vi "CANOpen SDOs - startup.vi"(8 "error in (no error)":errorcluster, 11 "Node Ptr":T2 format="%.0x") -> (0 "error out":errorcluster)   [LabVIEW 2013, in "CANOpen Addon Custom Device.lvlib"]
uses:
  CANOpen Addon Custom Device.lvlib
  <vilib>/NI Veristand/Custom Device API/Custom Device Item Ref.ctl
  SubVIs/CANOpen_SDO data format.ctl
  Shared Code/CANOpen_SDO Settings.ctl
  Shared Code/CANOpen Addon GUID Lookup Global.vi
  <vilib>/NI Veristand/Custom Device API/Get Item Property (Variant).vi
  <vilib>/NI Veristand/Custom Device API/Custom Device API.lvlib
panel:
  in  "Display format":T1
  out "SDOs":i32(listbox)
  in  "SHDocVw.IWebBrowser2":refnum<k7>(container)
  in  "Header":cluster{"Section Name":string}={"Section Name"="SDOs"}
  in  "Description":string
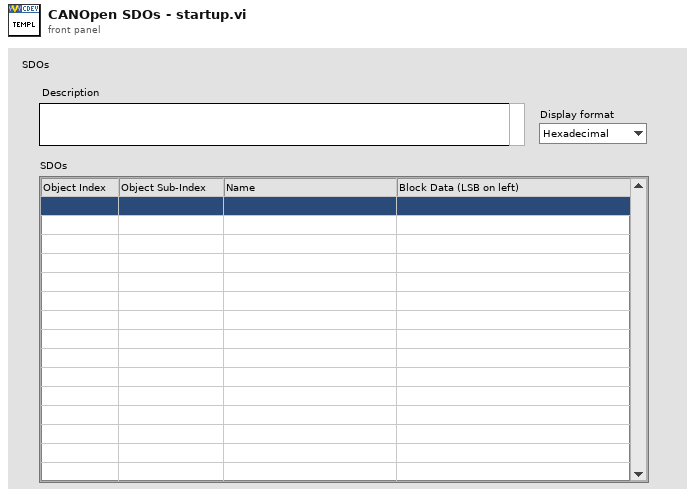
[diagram p1: front panel]
types:
  T1 = typedef "CANOpen Addon Custom Device.lvlib/CANOpen_SDO data format.ctl" = enum16{"Hexadecimal", "Decimal"}
  T2 = typedef "Custom Device API.lvlib/Custom Device Item Ref.ctl" = u64
  T3 = typedef "CANOpen Addon Custom Device.lvlib/CANOpen_SDO Settings.ctl" = cluster{"Object Index":u16, "Sub-Index (0)":u8, "Block Data":u8[], "Name":string}
  T4 = typedef "Custom Device API.lvlib/Custom Device Commands.ctl" = enum16{"Default", "Item renamed", "Shutdown", "Dynamic button pressed"}
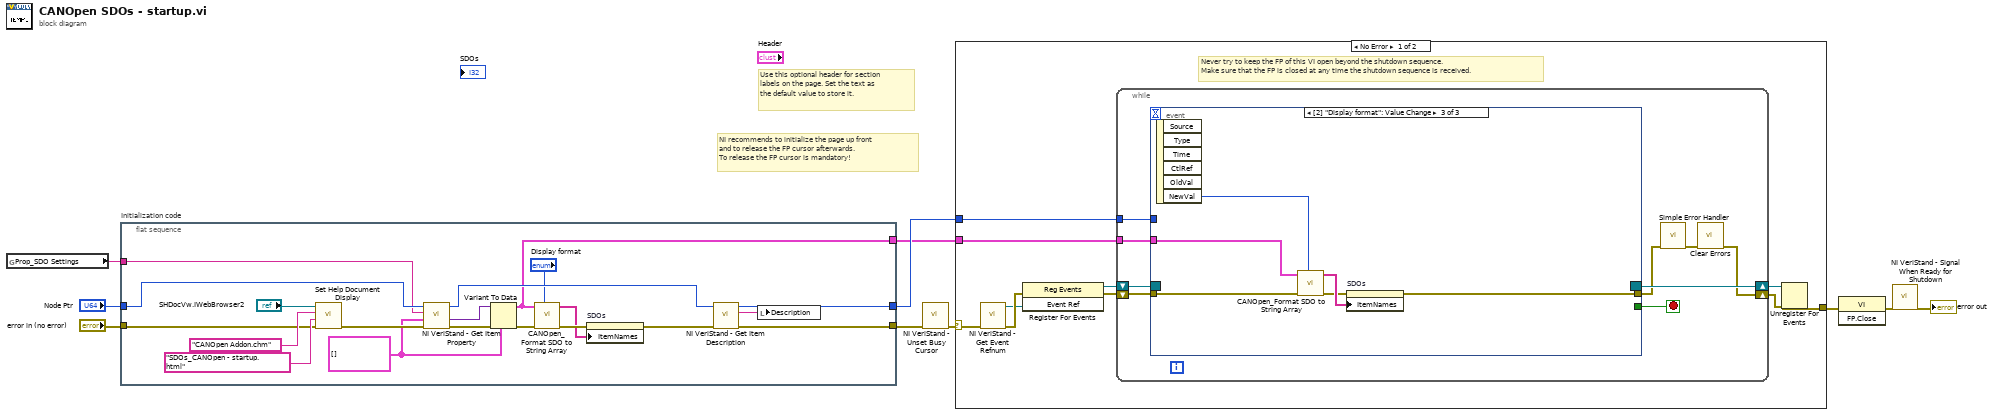
[diagram p0: block diagram]
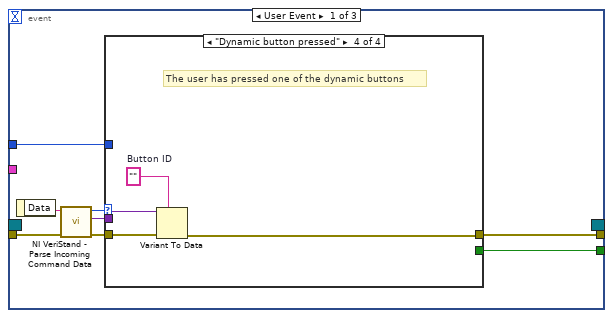
[diagram p2: hidden frame]
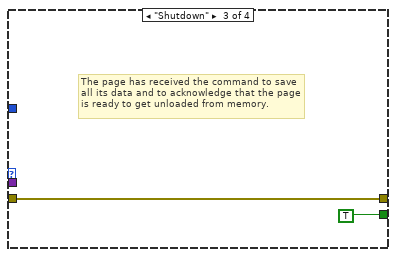
[diagram p5: hidden frame]
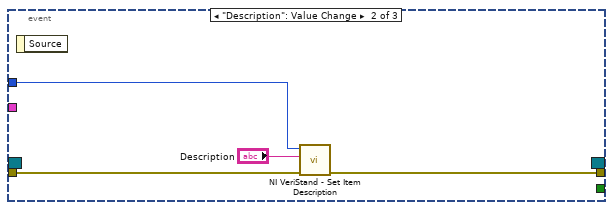
[diagram p6: hidden frame]
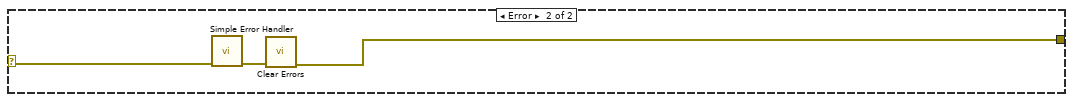
[diagram p7: hidden frame]
diagram:
  # "Use this optional header for section labels on the page. Set the text as the default value to store it."
  # "NI recommends to initialize the page up front\nand to release the FP cursor afterwards.\nTo release the FP cursor is mandatory!"
  n1 = global read "CANOpen Addon GUID Lookup Global.vi" "Prop_SDO Settings"() -> (w2:string)
  n2 = flat-sequence "Initialization code" {
    tunnel: "error in (no error)" -> [w26]
    tunnel: "Node Ptr" -> [w24]
    tunnel: [w13] -> w6
    tunnel: [w12] -> w3
    tunnel: w2 -> [w22]
    tunnel: [w11] -> w1
    frame #0 {
      w19 = T3[] [] ("SDO Parameters")
      n3 = call "Set Help Document Display.vi"("error in (no error)"=w26, "HTML File"="SDOs_CANOpen - startup.html", "Main CHM File"="CANOpen Addon.chm", "SHDocVw.IWebBrowser2"="SHDocVw.IWebBrowser2") -> ("error out"=w25:errorcluster)  [unwired: 7 in]
      n4 = call-poly <vilib>:"NI VeriStand - Get Item Property.vi"("error in (no error)"=w25, "Default Value"=w19, "Property Name"=w22, "Item Ref in"=w24) -> ("error out"=w21:errorcluster, "Value"=w20:variant, "Item Ref out"=w23:T2)  [unwired: 4 in, 1 out]
      n5 = Variant To Data(error in=w21, type=w19, Variant=w20) -> (data=w11:T3[], error out=w18:errorcluster)
      n6 = call "CANOpen_Format SDO to String Array.vi"("Format"="Display format", "error in (no error)"=w18, "SDO Parameters"=w11) -> ("error out"=w17:errorcluster, "Array"=w15:string[][])  [unwired: 7 in]
      n7 = property on="SDOs" class="MCListbox (strict)"(error in=w17, "ItemNames"=w15) -> (error out=w16:errorcluster)  [unwired: 1 in, 1 out]
      n8 = call <vilib>:"NI VeriStand - Get Item Description.vi"("error in (no error)"=w16, "Item Ref in"=w23) -> ("error out"=w13:errorcluster, "Description"=w30:string, "Item Ref out"=w12:T2)  [unwired: 7 out]
      n9 = local write "Description"(w30) -> ()
    }
  }
  n10 = call <vilib>:"NI VeriStand - Unset Busy Cursor.vi"("error in (no error)"=w6) -> ("error out"=w5:errorcluster)  [unwired: 10 out]
  n11 = case shown="No Error" w5 {
    selector: w5 -> [w32 w78]
    tunnel: [w37 w76] -> w10
    tunnel: w3 -> [w33 _]
    tunnel: w1 -> [w31 _]
    frame No Error {
      # "Never try to keep the FP of this VI open beyond the shutdown sequence.\nMake sure that the FP is closed at any time the shutdown sequence is received."
      n12 = call <vilib>:"NI VeriStand - Get Event Refnum.vi"("error in (no error)"=w32) -> ("error out"=w40:errorcluster, "Event Ref"=w36:refnum<user-event>)  [unwired: 9 out]
      n13 = register-events(error in=w40, w36) -> (reference out=w34:refnum<event-registration>, error out=w35:errorcluster)  [unwired: 1 in]
      n14 = while {
        tunnel: w33 -> [w45]
        shift-right: [w42] -> w38
        shift-left: w35 -> [w48]
        shift-right: [w49] -> w39
        shift-left: w34 -> [w47]
        tunnel: w31 -> [w41]
        stop <- w46 stop-if-true
        n15 = event shown="[2] \"Display format\": Value Change" {
          selector: w47 -> [_ _ _]
          dyn-events: [_ _ _] -> w49
          timeout: _ -> [_ _ _]
          tunnel: w48 -> [w57 w68 w71]
          tunnel: [w53 _ _] -> w46
          tunnel: [w52 w67 w70] -> w44
          tunnel: w45 -> [w51 w69 _]
          tunnel: w41 -> [_ _ w73]
          event User Event {
            n16 = event-data() -> ("Data"=w56:string)  [unwired: 1 out]
            n17 = call <vilib>:"NI VeriStand - Parse Incoming Command Data.vi"("error in (no error)"=w57, "Incoming data"=w56) -> ("error out"=w55:errorcluster, "Outgoing data"=w50:variant, "Action"=w54:T4)  [unwired: 7 out]
            n18 = case shown="\"Dynamic button pressed\"" w54 {
              tunnel: w55 -> [w58 w59 w60 w65]
              tunnel: [_ _ TRUE _] -> w53
              tunnel: [w58 w59 w60 w62] -> w52
              tunnel: w51 -> [_ _ _ _]
              tunnel: w50 -> [_ _ _ w64]
              frame "Default", Default {
              }
              frame "Item renamed" {
              }
              frame "Shutdown" {
                # "The page has received the command to save all its data and to acknowledge that the page is ready to get unloaded from memory."
              }
              frame "Dynamic button pressed" {
                w63 = ""  # Button ID
                # "The user has pressed one of the dynamic buttons"
                n19 = Variant To Data(error in=w65, type=w63, Variant=w64) -> (error out=w62:errorcluster)  [unwired: 1 out]
              }
            }
          }
          event "Description": Value Change {
            n20 = event-data() -> ()  [unwired: 2 out]
            n21 = call <vilib>:"NI VeriStand - Set Item Description.vi"("error in (no error)"=w68, "Description"="Description", "Item Ref in"=w69) -> ("error out"=w67:errorcluster)  [unwired: 8 out]
          }
          event Value Change {
            n22 = event-data() -> ("NewVal"=w72:T1)  [unwired: 6 out]
            n23 = call "CANOpen_Format SDO to String Array.vi"("Format"=w72, "error in (no error)"=w71, "SDO Parameters"=w73) -> ("error out"=w74:errorcluster, "Array"=w75:string[][])  [unwired: 7 in]
            n24 = property on="SDOs" class="MCListbox (strict)"(error in=w74, "ItemNames"=w75) -> (error out=w70:errorcluster)  [unwired: 1 in, 1 out]
          }
        }
        n25 = call <vilib>:"Simple Error Handler.vi"("error in (no error)"=w44) -> ("error out"=w43:errorcluster)  [unwired: 1 in, 7 out]
        n26 = call <vilib>:"Clear Errors.vi"("error in (no error)"=w43) -> ("error out"=w42:errorcluster)  [unwired: 6 out]
      }
      n27 = Unregister For Events(event registration refnum=w39, error in=w38) -> (error out=w37:errorcluster)
    }
    frame Error {
      n28 = call <vilib>:"Simple Error Handler.vi"("error in (no error)"=w78) -> ("error out"=w77:errorcluster)  [unwired: 1 in, 7 out]
      n29 = call <vilib>:"Clear Errors.vi"("error in (no error)"=w77) -> ("error out"=w76:errorcluster)  [unwired: 6 out]
    }
  }
  n30 = invoke class="VI" method="FP.Close"(error in=w10) -> (error out=w9:errorcluster)  [unwired: 2 in, 2 out]
  n31 = call <vilib>:"NI VeriStand - Signal When Ready for Shutdown.vi"("error in (no error)"=w9) -> ("error out"=→"error out":errorcluster)  [unwired: 10 out]
